vi "niFPGA Zero-Order Hold_m.vi"   [LabVIEW 2017]
doc: "Samples an input signal and holds it for a specified number of calls to the VI. The data type you wire to <B>input</B> determines the <B>output</B> data type."
uses:
  <vilib>/rvi/Analysis/common/FxpNativeNode/niFpgaFxpNative.xnode
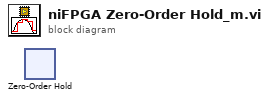
[diagram p0: block diagram]
diagram:
  n1 = xnode ("Zero-Order Hold")() -> ()  [unwired: 3 in, 1 out]
